vi "Test PLL.vi"(8 "error in (no error)":errorcluster, 11 "Lockin.DAQ":refnum<class "Lockin.DAQ.lvclass">) -> (0 "error out":errorcluster, 3 "Lockin.DAQ out":refnum<class "Lockin.DAQ.lvclass">)   [LabVIEW 2016, in "Lockin.DAQ.lvclass"]
uses:
  Lockin.DAQ.lvclass
  Typedefs/Sampling.ctl
  Typedefs/AO-cluster.ctl
  Instrument.Lockinl.UI/Typedefs/AO Channel--Cluster.ctl
  Typedefs/Function-enum.ctl
  Typedefs/REF-cluster.ctl
  Instrument.Lockinl.UI/Typedefs/REF Channel--Cluster.ctl
  Lockin.DAQ.lvclass/Lockin.DAQ.ctl
  Instrument.Lockinl.UI/Instrument.Lockin.UI.lvclass
panel:
  in  "index":i32
  in  "Configuration.Channels: REF":T1 {"Order" min=1; "TC" min=0.0001 format="%#_3p"; "Phase" format="%.3g"; "Frequency" min=0.0001 max=10000.0 format="%.3g"}
  in  "Channels: AO":T3 {"REF.Ch 2" items=["1"]; "REF.Ch 1" items=["1"]; "Phase" format="%.3g"; "Frequency" min=0.0001 max=10000.0 format="%.3g"; "Offset" format="%.3p"; "Amplitude" min=0.0 max=10.0 format="%.3p"}
  in  "Enum":enum16{"X", "Y", "R", "Theta", "Mean"}(ring)
  out "Waveform Chart":dbl[][](graph)=[[-0.22911635604378638]]
  out "Waveform Graph":waveform(dbl)[](graph)=[{"t0"=timestamp(0 s since 1904-01-01), "dt"=1.0, "Y"=[]}, {"t0"=timestamp(0 s since 1904-01-01), "dt"=1.0, "Y"=[]}]
  in  "sampling":T6={"Fs"=204789.0, "#s"=15753}
  in  "stop":bool
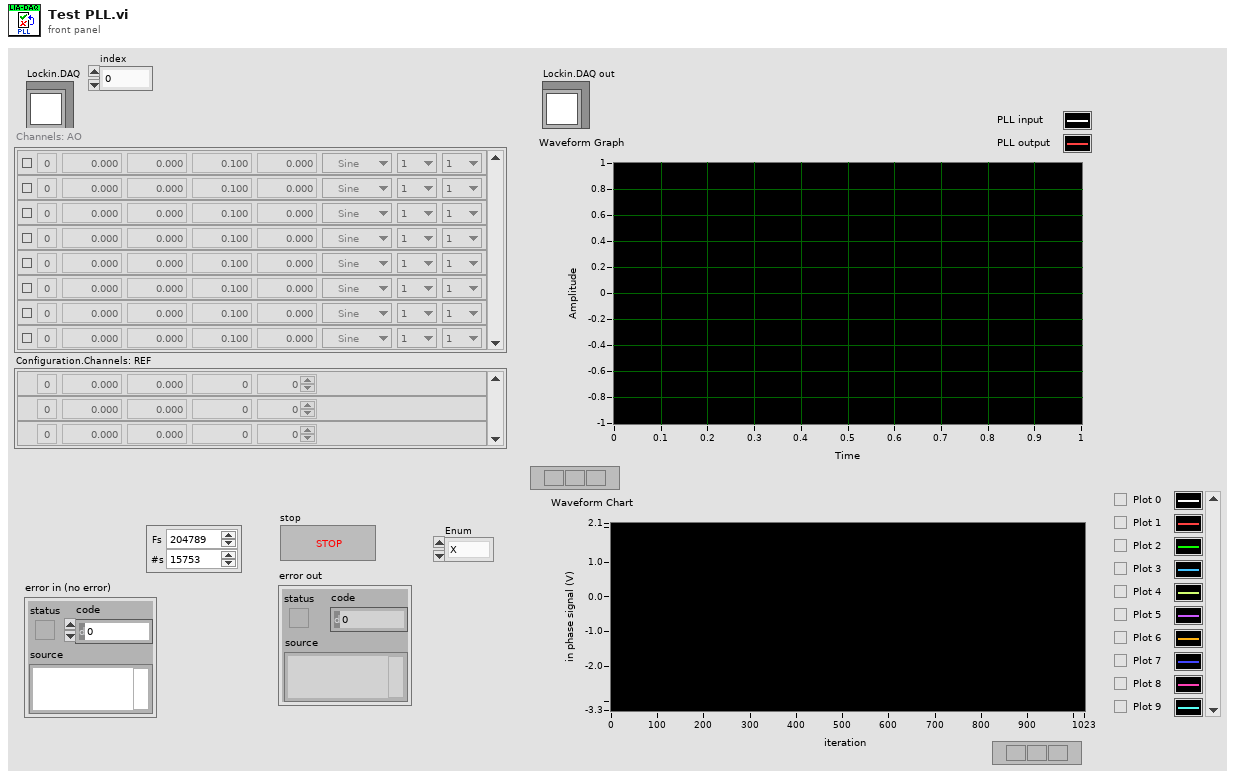
[diagram p1: front panel]
types:
  T1 = typedef "Lockin.DAQ.lvclass/REF-cluster.ctl" = T2[]
  T2 = typedef "Instrument.Lockin.UI.lvclass/REF Channel--Cluster.ctl" = cluster{"Channel":i32, "Frequency":dbl, "Phase":dbl, "TC":dbl, "Order":i32}
  T3 = typedef "Lockin.DAQ.lvclass/AO-cluster.ctl" = T4[]
  T4 = typedef "Instrument.Lockin.UI.lvclass/AO Channel--Cluster.ctl" = cluster{"Channel":i32, "Amplitude":dbl, "Offset":dbl, "Frequency":dbl, "Phase":dbl, "Function":T5, "Sweeping?":bool, "REF.Ch 1":u16, "REF.Ch 2":u16}
  T5 = typedef "Lockin.DAQ.lvclass/Function-enum.ctl" = enum16{"Sine", "Triangle", "Square"}
  T6 = typedef "Lockin.DAQ.lvclass/Sampling.ctl" = cluster{"Fs":dbl, "#s":i32}
  T7 = typedef "Lockin.DAQ.lvclass/Results--Cluster.ctl" = cluster{"Time Stamp":timestamp, "Results":dbl[][]}
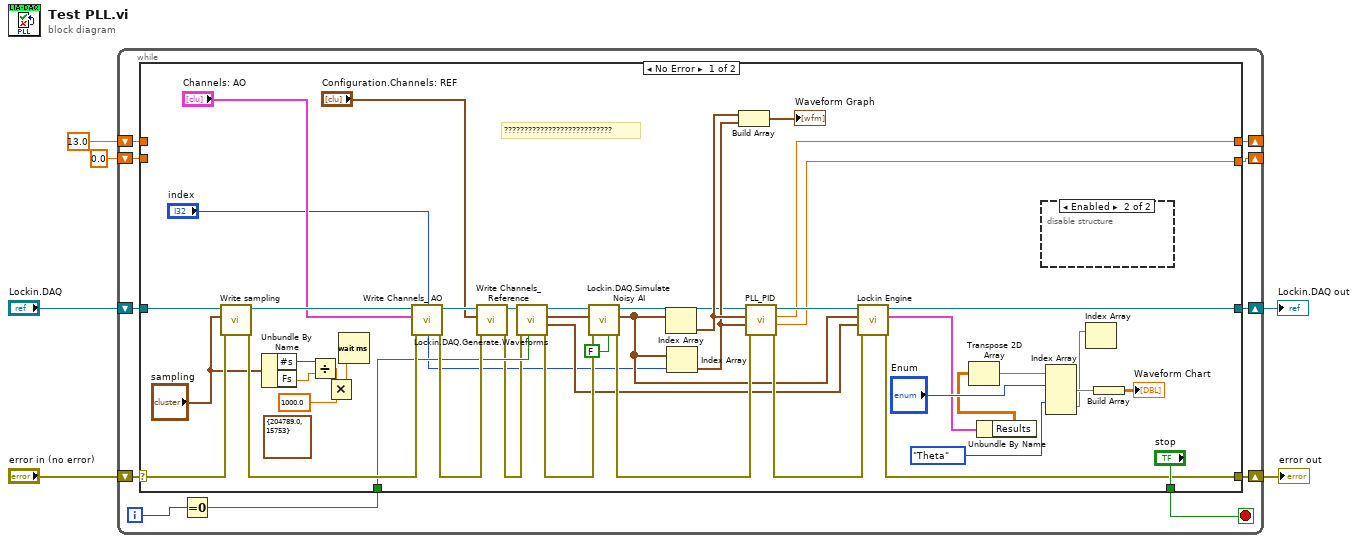
[diagram p0: block diagram]
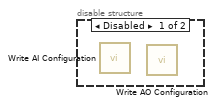
[diagram p2: hidden frame]
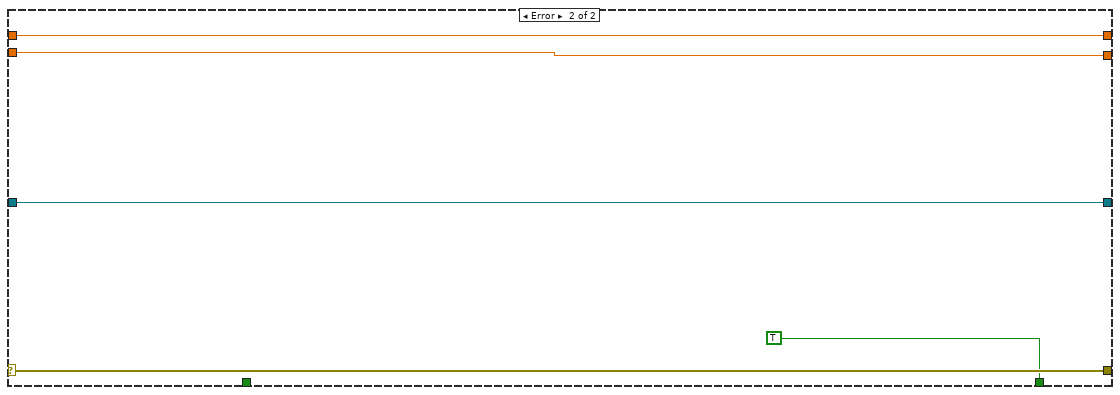
[diagram p3: hidden frame]
diagram:
  n1 = while {
    shift-right: [w16] -> w5
    shift-left: "error in (no error)" -> [w17]
    shift-right: [w14] -> w3
    shift-left: "Lockin.DAQ" -> [w15]
    shift-right: [w10] -> _
    shift-left: 13.0 -> [w8]
    shift-right: [w9] -> _
    shift-left: 0.0 -> [w7]
    i -> [w12]
    stop <- w11 stop-if-true
    n2 = Equal To 0?(x=w12) -> (x = 0?=w13:bool)
    n3 = case shown="No Error" w17 {
      selector: w17 -> [w60 w66]
      tunnel: [w27 w66] -> w16
      tunnel: [w33 w65] -> w14
      tunnel: w15 -> [w61 w65]
      tunnel: w13 -> [w55 _]
      tunnel: ["stop" TRUE ("stop")] -> w11
      tunnel: [w25 w62] -> w10
      tunnel: [w24 w63] -> w9
      tunnel: w8 -> [_ w62]
      tunnel: w7 -> [_ w63]
      frame No Error {
        (unwired) T6 {"Fs"=204789.0, "#s"=15753} ("sampling")
        # "???????????????????????????"
        n4 = call "Write sampling.vi"("error in (no error)"=w60, "sampling"="sampling", "Lockin.DAQ"=w61) -> ("error out"=w56:errorcluster, "Lockin.DAQ out"=w57:refnum<class "Lockin.DAQ.lvclass">)  [unwired: 7 in]
        n5 = Unbundle By Name("sampling") -> ("#s"=w47:i32, "Fs"=w46:dbl)
        n6 = Divide(x=w47, y=w46) -> (x/y=w45:dbl)
        n7 = Multiply(x=w45, y=1000.0) -> (x*y=w44:dbl)
        n8 = Wait (ms)(milliseconds to wait=w44) -> ()  [unwired: 1 out]
        n9 = call "Write Channels_ AO.vi"("error in (no error)"=w56, "Channels: AO"="Channels: AO", "Lockin.DAQ"=w57) -> ("error out"=w58:errorcluster, "Lockin.DAQ out"=w59:refnum<class "Lockin.DAQ.lvclass">)  [unwired: 7 in]
        n10 = call "Write Channels_ Reference.vi"("error in (no error)"=w58, "Configuration.Channels: REF"="Configuration.Channels: REF", "Lockin.DAQ"=w59) -> ("error out"=w54:errorcluster, "Lockin.DAQ out"=w53:refnum<class "Lockin.DAQ.lvclass">)  [unwired: 7 in]
        n11 = call "Lockin.DAQ.Generate.Waveforms.vi"("Reset?"=w55, "error in (no error)"=w54, "Lockin.DAQ"=w53) -> ("error out"=w42:errorcluster, "REF []"=w23:waveform(dbl)[], "AO []"=w43:waveform(dbl)[], "Lockin.DAQ"=w40:refnum<class "Lockin.DAQ.lvclass">)  [unwired: 5 in]
        n12 = call "Lockin.DAQ.Simulate Noisy AI.vi"("Simulate Waveguide [T]"=FALSE, "error in (no error)"=w42, "AO []"=w43, "Lockin.DAQ in"=w40) -> ("error out"=w29:errorcluster, "Noisy AI []"=w21:waveform(dbl)[], "Lockin.DAQ out"=w30:refnum<class "Lockin.DAQ.lvclass">)  [unwired: 5 in]
        n13 = Index Array(array=w21) -> (element=w50:waveform(dbl))  [unwired: 1 in]
        n14 = Index Array(array=w21, index="index") -> (element=w49:waveform(dbl))
        n15 = Build Array(w50, w49) -> (→"Waveform Graph":waveform(dbl)[])
        n16 = call "PLL_PID.vi"("error in (no error)"=w29, "Oscillator []"=w49, "Target []"=w50, "LockinDAQ in"=w30) -> ("error out"=w28:errorcluster, "phase output (°)"=w24:dbl, "frequency output (Hz)"=w25:dbl, "LockinDAQ out"=w26:refnum<class "Lockin.DAQ.lvclass">)  [unwired: 4 in]
        n17 = call "Lockin Engine.vi"("error in (no error)"=w28, "REF Waveforms"=w23, "AI Waveforms"=w21, "Lockin.DAQ"=w26) -> ("error out"=w27:errorcluster, "Averaged Results (X,Y,R,Theta,Mean)"=w35:T7, "Lockin.DAQ"=w33:refnum<class "Lockin.DAQ.lvclass">)  [unwired: 4 in, 1 out]
        n18 = Unbundle By Name(w35) -> ("Results"=w34:dbl[][])
        n19 = Transpose 2D Array(2D array=w34) -> (transposed array=w36:dbl[][])
        n20 = disable-structure shown="Enabled" {
          frame Disabled {
            n21 = call "Write AI Configuration.vi"() -> ()  [unwired: 10 in, 2 out]
            n22 = call "Write AO Configuration.vi"() -> ()  [unwired: 10 in, 2 out]
          }
          frame Enabled {
          }
        }
        n23 = Index Array(array=w36, index (row) #1="Enum", index (row) #2=enum16{"X", "Y", "R", "Theta", "Mean"}."Theta" ("Enum")) -> (element #1=w37:dbl[], element #2=w31:dbl[])  [unwired: 2 in]
        n24 = Index Array(array=w31) -> ()  [unwired: 1 in, 1 out]
        n25 = Build Array(w37) -> (→"Waveform Chart":dbl[][])
      }
      frame Error {
      }
    }
  }
  "error out" <- w5
  "Lockin.DAQ out" <- w3
